vi "Configure Output Waveform.vi"(0 "VISA resource name":refnum<visa-resource-name>, 1 "User-Specified Output Waveform Name":string, 2 "User-Specified Triggered Output Waveform Name":string, 5 "Output Waveform Type (0: Sinusoid)":u16(ring) items=["Sinusoid", "Square", "Clipped Sinusoid", "User Specified"], 7 "Output Waveform Mode (0: Fix)":u16(ring) items=["Fixed", "Step", "Pulse", "List"], 9 "Triggered Output Waveform Type (0: Sinusoid)":u16(ring) items=["Sinusoid", "Square", "Clipped Sinusoid", "User Specified"], 11 "error in (no error)":errorcluster, 12 "Clipping Type (0: Peak)":u16(ring) items=["Peak", "Total Harmonic Distortion"], 13 "Clipping Level (20 %)":dbl=20.0 format="%#.4g") -> (4 "VISA resource name out":refnum<visa-resource-name>, 15 "error out":errorcluster)   [LabVIEW 2020, in "Agilent 681x Series.lvlib"]
doc: "Configures the output shape properties."
uses:
  <instrlib>/Agilent 681x Series/Agilent 681x Series.lvlib
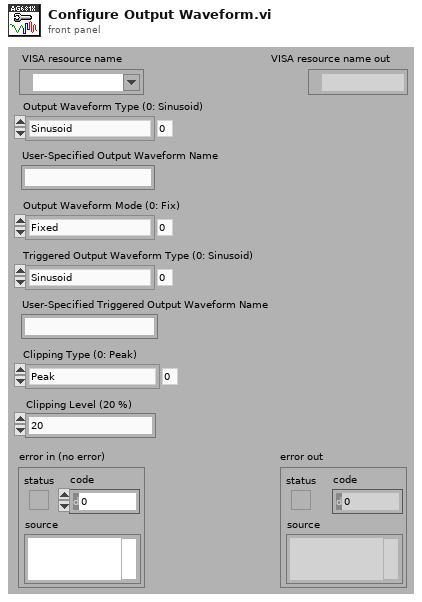
[diagram p1: front panel]
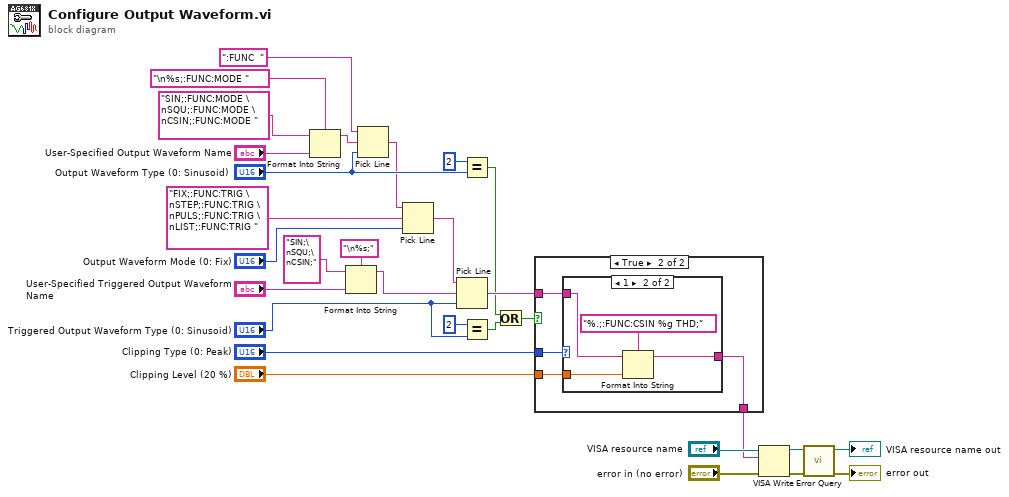
[diagram p0: block diagram]
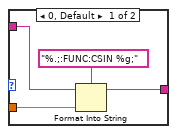
[diagram p3: hidden frame]
diagram:
  n1 = Format Into String(format string="\n%s;:FUNC:MODE ", initial string="SIN;:FUNC:MODE \nSQU;:FUNC:MODE \nCSIN;:FUNC:MODE " ("multi-line string"), "User-Specified Output Waveform Name") -> (resulting string=w4:string)  [unwired: 1 in, 1 out]
  n2 = Format Into String(format string="\n%s;", initial string="SIN;\nSQU;\nCSIN;" ("multi-line string"), "User-Specified Triggered Output Waveform Name") -> (resulting string=w13:string)  [unwired: 1 in, 1 out]
  n3 = Pick Line(string ("")=":FUNC  ", multi-line string=w4, line index="Output Waveform Type (0: Sinusoid)") -> (output string=w1:string)
  n4 = Pick Line(string ("")=w1, multi-line string="FIX;:FUNC:TRIG \nSTEP;:FUNC:TRIG \nPULS;:FUNC:TRIG \nLIST;:FUNC:TRIG ", line index="Output Waveform Mode (0: Fix)") -> (output string=w22:string)
  n5 = Pick Line(string ("")=w22, multi-line string=w13, line index="Triggered Output Waveform Type (0: Sinusoid)") -> (output string=w19:string)
  n6 = Equal?(x=u16 2, y="Output Waveform Type (0: Sinusoid)") -> (x = y?=w7:bool)
  n7 = Equal?(x=u16 2, y="Triggered Output Waveform Type (0: Sinusoid)") -> (x = y?=w8:bool)
  n8 = Or(x=w7, y=w8) -> (x .or. y?=w9:bool)
  n9 = case shown="True" w9 {
    tunnel: "Clipping Type (0: Peak)" -> [_ w35]
    tunnel: "Clipping Level (20 %)" -> [_ w34]
    tunnel: w19 -> [w31 w33]
    tunnel: [w31 w32] -> w18
    frame False {
    }
    frame True {
      n10 = case shown="1" w35 {
        tunnel: w34 -> [w39 w42]
        tunnel: w33 -> [w38 w40]
        tunnel: [w36 w43] -> w32
        frame 0, Default {
          n11 = Format Into String(format string="%.;:FUNC:CSIN %g;", initial string=w38, w39) -> (resulting string=w36:string)  [unwired: 1 in, 1 out]
        }
        frame 1 {
          n12 = Format Into String(format string="%.;:FUNC:CSIN %g THD;", initial string=w40, w42) -> (resulting string=w43:string)  [unwired: 1 in, 1 out]
        }
      }
    }
  }
  n13 = VISA Write(VISA resource name="VISA resource name", write buffer=w18, error in (no error)="error in (no error)") -> (VISA resource name out=w28:refnum<visa-resource-name>, error out=w27:errorcluster)  [unwired: 1 out]
  n14 = call <instrlib>:"Error Query.vi"("error in (no error)"=w27, "VISA resource name"=w28) -> ("error out"=→"error out":errorcluster, "VISA resource name out"=→"VISA resource name out":refnum<visa-resource-name>)  [unwired: 6 in, 2 out]
